vi "SVPO Integration (1 CH DBL Array) with IC.vi"(6 "reset filters":bool, 8 "initial conditions":T1 {"filter state"."initial highpass filter state" format="%.2f"; "filter state"."initial integration fiter state"."y(n-2) state" format="%.2f"; "filter state"."initial integration fiter state"."x(n-2) state" format="%.2f"; "filter state"."initial integration fiter state"."y(n-1) state" format="%.2f"; "filter state"."initial integration fiter state"."x(n-1) state" format="%.2f"; "filter coefficents"."highpass filter coefficients"."Forward Coefficients" format="%.2f"; "filter coefficents"."highpass filter coefficients"."Reverse Coefficients" format="%.2f"; "filter coefficents"."integration filter coefficients"."alpha" format="%.2f"; "filter coefficents"."integration filter coefficients"."gamma" format="%.2f"; "filter coefficents"."integration filter coefficients"."beta" format="%.2f"}, 9 "highpass cutoff frequency [Hz]":dbl=1.0 format="%.2f", 10 "sampling rate [Hz]":dbl=1.0, 11 "scaled signal [EU]":dbl[](array[numeric])) -> (0 "final conditions":T1 {"filter state"."initial highpass filter state" format="%.2f"; "filter state"."initial integration fiter state"."y(n-2) state" format="%.2f"; "filter state"."initial integration fiter state"."x(n-2) state" format="%.2f"; "filter state"."initial integration fiter state"."y(n-1) state" format="%.2f"; "filter state"."initial integration fiter state"."x(n-1) state" format="%.2f"; "filter coefficents"."highpass filter coefficients"."Forward Coefficients" format="%.2f"; "filter coefficents"."highpass filter coefficients"."Reverse Coefficients" format="%.2f"; "filter coefficents"."integration filter coefficients"."alpha" format="%.2f"; "filter coefficents"."integration filter coefficients"."gamma" format="%.2f"; "filter coefficents"."integration filter coefficients"."beta" format="%.2f"}, 3 "integrated signal [EU*s]":dbl[](array[numeric]))   [LabVIEW 2017, in "SoundVib_Integration.lvlib"]
doc: "Converts acceleration to velocity or velocity to displacement using a time-domain waveform as the input. Wire data to the <B>scaled signal [EU]</B> input to determine the polymorphic instance to use or manually select the instance. This VI performs Single Integration only. You can pass the integrated signal [EU*s] output to the scaled signal [EU] input of second call to this VI to perform double integration."
uses:
  <vilib>/addons/Sound and Vibration/svt_Integration/SoundVib_Integration.lvlib
  <vilib>/addons/_NISVFA/_Shared subVIs/Controls/svc_Integration State.ctl
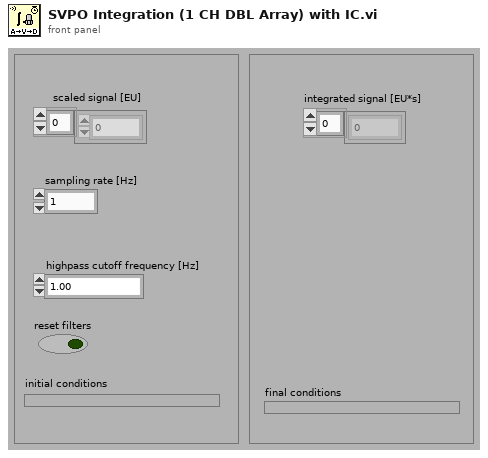
[diagram p1: front panel]
types:
  T1 = typedef "svc_Integration State.ctl" = cluster{"filter coefficents":cluster{"integration filter coefficients":cluster{"beta":dbl, "gamma":dbl, "alpha":dbl}, "highpass filter coefficients":cluster{"filter structure":enum32{"IIR 2nd Order", "IIR 4th Order"}, "Reverse Coefficients":dbl[], "Forward Coefficients":dbl[]}}, "filter state":cluster{"initial integration fiter state":cluster{"x(n-1) state":dbl, "y(n-1) state":dbl, "x(n-2) state":dbl, "y(n-2) state":dbl}, "initial highpass filter state":dbl[]}}
  T2 = cluster{"filter structure":enum32{"IIR 2nd Order", "IIR 4th Order"}, "Reverse Coefficients":dbl[], "Forward Coefficients":dbl[]}
  T3 = cluster{"x(n-1) state":dbl, "y(n-1) state":dbl, "x(n-2) state":dbl, "y(n-2) state":dbl}
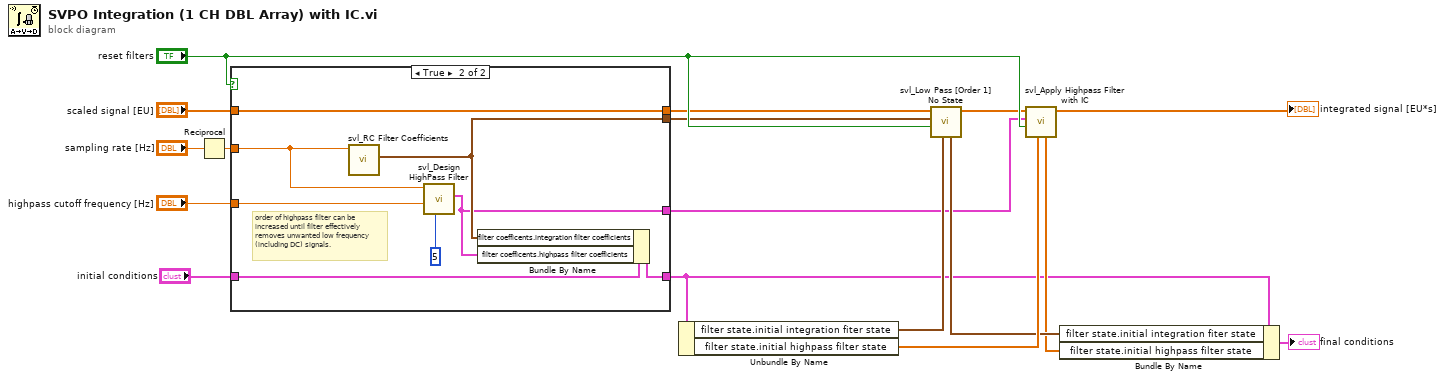
[diagram p0: block diagram]
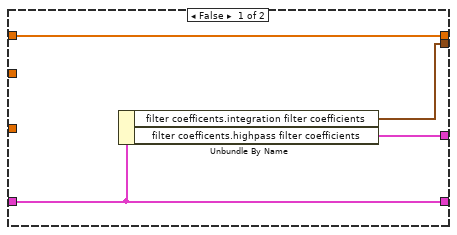
[diagram p2: hidden frame]
diagram:
  n1 = Reciprocal(x="sampling rate [Hz]") -> (1/x=w5:dbl)
  n2 = case shown="True" "reset filters" {
    tunnel: "scaled signal [EU]" -> [w21 w23]
    tunnel: [w21 w23] -> w4
    tunnel: "highpass cutoff frequency [Hz]" -> [_ w29]
    tunnel: [w19 w26] -> w11
    tunnel: [w20 w27] -> w10
    tunnel: "initial conditions" -> [w18 w24]
    tunnel: [w18 w25] -> w1
    tunnel: w5 -> [_ w22]
    frame False {
      n3 = Unbundle By Name(w18) -> ("filter coefficents.integration filter coefficients"=w20:cluster{"beta":dbl, "gamma":dbl, "alpha":dbl}, "filter coefficents.highpass filter coefficients"=w19:T2)
    }
    frame True {
      # "order of highpass filter can be\nincreased until filter effectively\nremoves unwanted low frequency\n(including DC) signals."
      n4 = call <vilib>:"svl_RC Filter Coefficients.vi"("dt"=w22) -> ("filter coefficients"=w27:cluster{"beta":dbl, "gamma":dbl, "alpha":dbl})  [unwired: 10 in]
      n5 = call <vilib>:"svl_Design HighPass Filter.vi"("highpass filter order"=5 ("order of filter can be\nincreased until filter\neffectively removes\nunwanted low\nfrequency (including\nDC) signals."), "highpass cutoff frequency"=w29, "dt"=w22) -> ("IIR Filter Cluster"=w26:T2)  [unwired: 7 in, 1 out]
      n6 = Bundle By Name(cluster=w24, "filter coefficents.integration filter coefficients"=w27, "filter coefficents.highpass filter coefficients"=w26) -> (w25:T1)
    }
  }
  n7 = Unbundle By Name(w1) -> ("filter state.initial integration fiter state"=w14:T3, "filter state.initial highpass filter state"=w15:dbl[])
  n8 = call <vilib>:"svl_Low Pass [Order 1] No State.vi"("state info in"=w14, "reset"="reset filters", "filter coefficients"=w10, "Input stream"=w4) -> ("filtered signal"=w9:dbl[], "state info out"=w13:T3)  [unwired: 6 in]
  n9 = call <vilib>:"svl_Apply Highpass Filter with IC.vi"("Initial Filter State"=w15, "reset"="reset filters", "filter coefficients"=w11, "signal [V]"=w9) -> ("filtered signal [EU]"=→"integrated signal [EU*s]":dbl[], "Final Filter State"=w12:dbl[])  [unwired: 5 in, 1 out]
  n10 = Bundle By Name(cluster=w1, "filter state.initial integration fiter state"=w13, "filter state.initial highpass filter state"=w12) -> (→"final conditions":T1)
